vi "TP_Calculate.vi"(8 "error in (no error)":errorcluster, 10 "t":dbl=-1.0, 11 "TrapezoidalProfile in":refnum<class "TrapezoidalProfile.lvclass">) -> (0 "error out":errorcluster, 2 "Output":T1, 3 "TrapezoidalProfile out":refnum<class "TrapezoidalProfile.lvclass">)   [LabVIEW 2018, in "TrapezoidalProfile.lvclass"]
doc: "Calculate the correct position and velocity for the profile at a time <b>t</b> where the beginning of the profile was at time t = 0.\n<b>t</b> Time since the beginning of the profile."
uses:
  TrapezoidalProfile.lvclass
  State.ctl
  TrapezoidalProfile.lvclass/TrapezoidalProfile.ctl
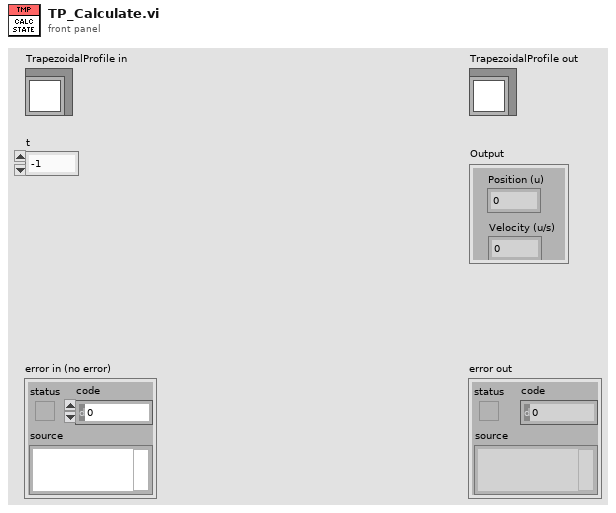
[diagram p1: front panel]
types:
  T1 = typedef "TrapezoidalProfile.lvclass/State.ctl" = cluster{"Position (u)":dbl, "Velocity (u/s)":dbl}
  T2 = typedef "TrapezoidalProfile.lvclass/Constraints.ctl" = cluster{"Max Velocity":dbl, "Max Accel":dbl}
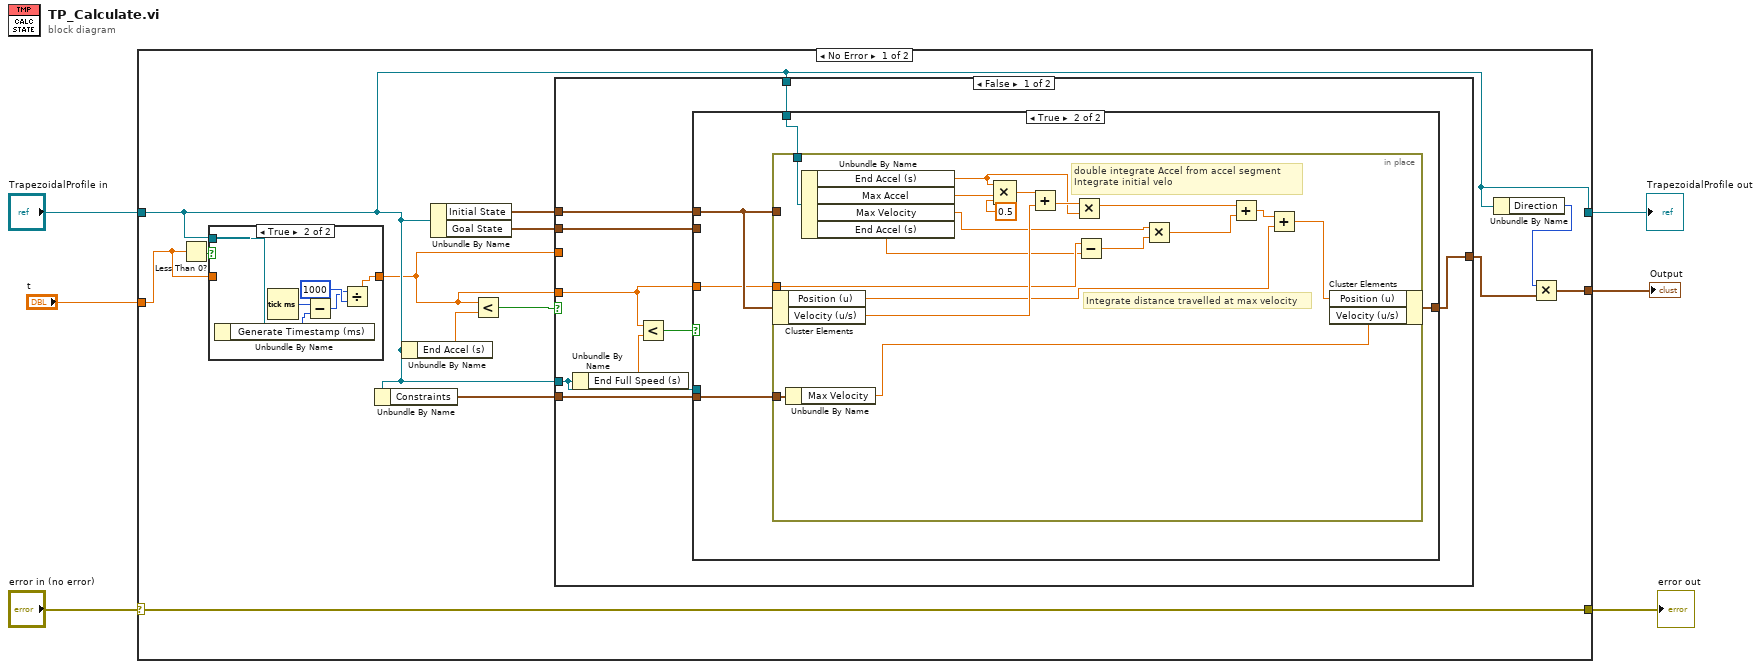
[diagram p0: block diagram]
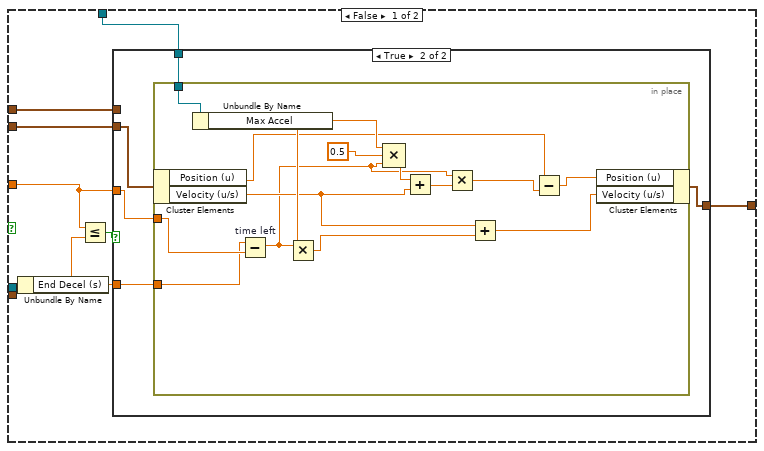
[diagram p3: hidden frame]
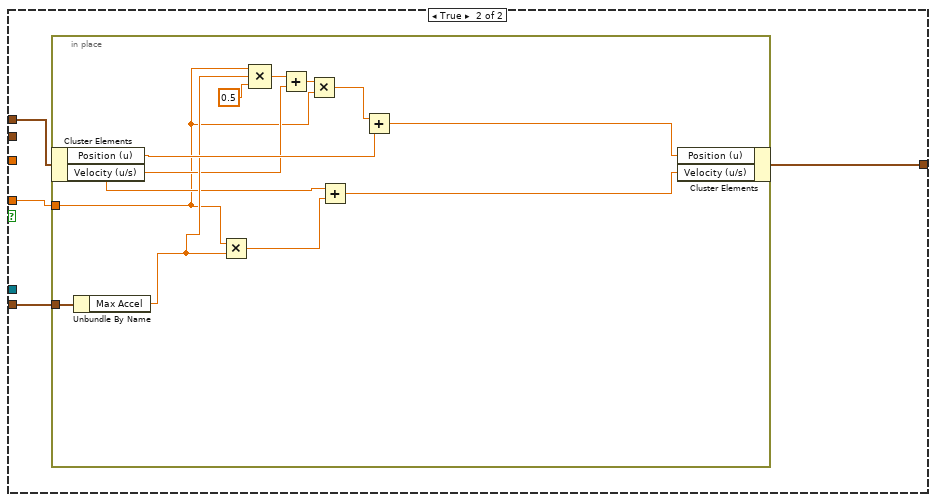
[diagram p5: hidden frame]
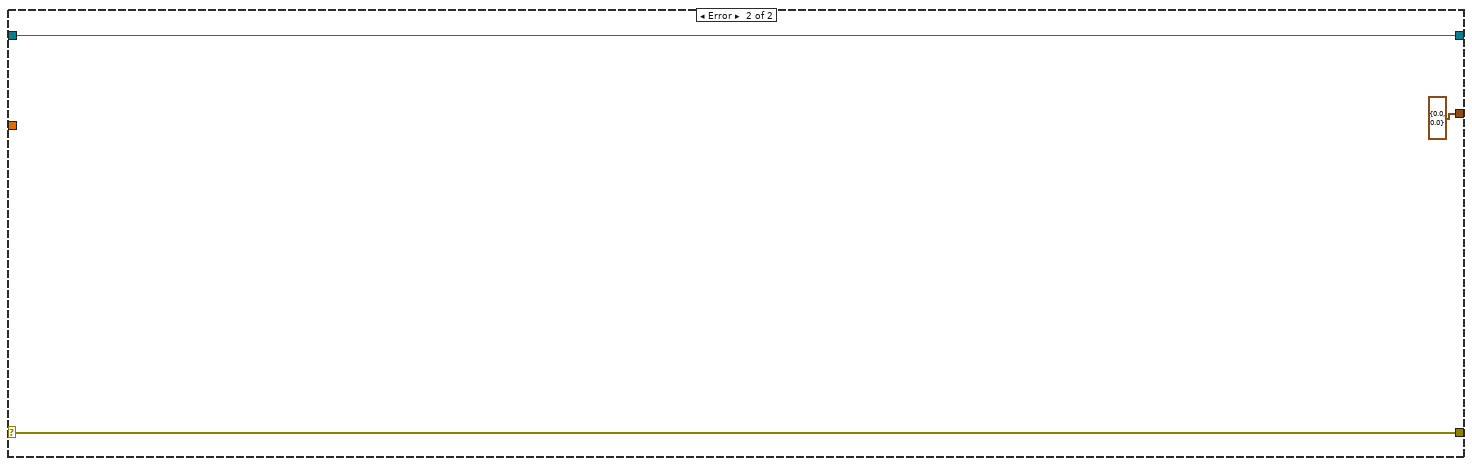
[diagram p6: hidden frame]
diagram:
  n1 = case shown="No Error" "error in (no error)" {
    selector: "error in (no error)" -> [w19 w105]
    tunnel: [w19 w105] -> w5
    tunnel: [w10 w104] -> w3
    tunnel: "TrapezoidalProfile in" -> [w10 w104]
    tunnel: "t" -> [w8 _]
    tunnel: [w11 T1 {"Position (u)"=0.0, "Velocity (u/s)"=0.0} ("Initial State")] -> w1
    frame No Error {
      n2 = Less Than 0?(x=w8) -> (x < 0?=w9:bool)
      n3 = case shown="True" w9 {
        tunnel: w10 -> [_ w26]
        tunnel: [w20 w23] -> w7
        tunnel: w8 -> [w20 _]
        frame False {
        }
        frame True {
          n4 = Unbundle By Name(w26) -> ("Generate Timestamp (ms)"=w24:u32)
          n5 = Tick Count (ms)() -> (millisecond timer value=w25:u32)
          n6 = Subtract(x=w25, y=w24) -> (x-y=w21:u32)
          n7 = Divide(x=w21, y=u32 1000 ("x")) -> (x/y=w23:dbl)
        }
      }
      n8 = Unbundle By Name(w10) -> ("Constraints"=w15:T2)
      n9 = Unbundle By Name(w10) -> ("End Accel (s)"=w18:dbl)
      n10 = Unbundle By Name(w10) -> ("Initial State"=w16:T1, "Goal State"=w14:T1)
      n11 = Less?(x=w7, y=w18) -> (x < y?=w17:bool)
      n12 = case shown="False" w17 {
        tunnel: w7 -> [_ _]
        tunnel: w16 -> [w33 w90]
        tunnel: w15 -> [w32 w89]
        tunnel: w7 -> [w31 w88]
        tunnel: [w28 w87] -> w12
        tunnel: w10 -> [w27 _]
        tunnel: w10 -> [w30 _]
        tunnel: w14 -> [w29 _]
        frame False {
          n13 = Unbundle By Name(w27) -> ("End Full Speed (s)"=w34:dbl)
          n14 = Less?(x=w31, y=w34) -> (x < y?=w35:bool)
          n15 = case shown="True" w35 {
            tunnel: w33 -> [w41 w67]
            tunnel: w32 -> [_ w68]
            tunnel: w31 -> [w37 w66]
            tunnel: w30 -> [w36 w65]
            tunnel: w29 -> [w43 _]
            tunnel: [w42 w64] -> w28
            tunnel: w27 -> [w39 _]
            frame False {
              n16 = Unbundle By Name(w39) -> ("End Decel (s)"=w38:dbl)
              n17 = Less Or Equal?(x=w37, y=w38) -> (x <= y?=w40:bool)
              n18 = case shown="True" w40 {
                tunnel: w43 -> [w44 w48]
                tunnel: [w44 w45] -> w42
                tunnel: w41 -> [_ _]
                tunnel: w38 -> [_ w49]
                tunnel: w37 -> [_ w47]
                tunnel: w36 -> [_ w46]
                frame False {
                }
                frame True {
                  n19 = in-place {
                    in-place-border: w49 -> [w62]
                    in-place-border: w47 -> [w63]
                    in-place-border: w46 -> [w61]
                    n20 = in-place-cluster #1(w48) -> ("Position (u)"=w50:dbl, "Velocity (u/s)"=w55:dbl)
                    n21 = Unbundle By Name(w61) -> ("Max Accel"=w58:dbl)
                    n22 = Subtract "time left"(x=w62, y=w63) -> (x-y=w53:dbl)
                    n23 = Multiply(x=w53, y=w58) -> (x*y=w60:dbl)
                    n24 = Compound Arithmetic op=MULTIPLY(w58, 0.5 ("value"), w53) -> (w56:dbl)
                    n25 = Add(x=w56, y=w55) -> (x+y=w54:dbl)
                    n26 = Multiply(x=w53, y=w54) -> (x*y=w51:dbl)
                    n27 = Add(x=w55, y=w60) -> (x+y=w59:dbl)
                    n28 = Subtract(x=w50, y=w51) -> (x-y=w52:dbl)
                    n29 = in-place-cluster #1("Position (u)"=w52, "Velocity (u/s)"=w59) -> (w45:T1)
                  }
                }
              }
            }
            frame True {
              n30 = in-place {
                in-place-border: w68 -> [w86]
                in-place-border: w67 -> [_]
                in-place-border: w66 -> [w77]
                in-place-border: w65 -> [w84]
                # "Integrate distance travelled at max velocity"
                # "double integrate Accel from accel segment\nIntegrate initial velo"
                n31 = in-place-cluster #2(w67) -> ("Position (u)"=w71:dbl, "Velocity (u/s)"=w81:dbl)
                n32 = Unbundle By Name(w86) -> ("Max Velocity"=w85:dbl)
                n33 = Unbundle By Name(w84) -> ("End Accel (s)"=w69:dbl, "Max Accel"=w79:dbl, "Max Velocity"=w78:dbl, "End Accel (s)"=w76:dbl)
                n34 = Compound Arithmetic op=MULTIPLY(w69, w79, 0.5 ("value")) -> (w82:dbl)
                n35 = Add(x=w82, y=w81) -> (x+y=w80:dbl)
                n36 = Multiply(x=w80, y=w69) -> (x*y=w74:dbl)
                n37 = Subtract(x=w77, y=w76) -> (x-y=w75:dbl)
                n38 = Multiply(x=w78, y=w75) -> (x*y=w73:dbl)
                n39 = Add(x=w74, y=w73) -> (x+y=w72:dbl)
                n40 = Add(x=w72, y=w71) -> (x+y=w70:dbl)
                n41 = in-place-cluster #2("Position (u)"=w70, "Velocity (u/s)"=w85) -> (w64:T1)
              }
            }
          }
        }
        frame True {
          n42 = in-place {
            in-place-border: w89 -> [w101]
            in-place-border: w88 -> [w92]
            n43 = in-place-cluster #3(w90) -> ("Position (u)"=w98:dbl, "Velocity (u/s)"=w94:dbl)
            n44 = Unbundle By Name(w101) -> ("Max Accel"=w97:dbl)
            n45 = Multiply(x=w92, y=w97) -> (x*y=w99:dbl)
            n46 = Compound Arithmetic op=MULTIPLY(w92, w97, 0.5 ("value")) -> (w95:dbl)
            n47 = Add(x=w95, y=w94) -> (x+y=w93:dbl)
            n48 = Multiply(x=w93, y=w92) -> (x*y=w91:dbl)
            n49 = Add(x=w94, y=w99) -> (x+y=w102:dbl)
            n50 = Add(x=w91, y=w98) -> (x+y=w100:dbl)
            n51 = in-place-cluster #3("Position (u)"=w100, "Velocity (u/s)"=w102) -> (w87:T1)
          }
        }
      }
      n52 = Unbundle By Name(w10) -> ("Direction"=w13:i32)
      n53 = Multiply(x=w13, y=w12) -> (x*y=w11:T1)
    }
    frame Error {
    }
  }
  "error out" <- w5
  "TrapezoidalProfile out" <- w3
  "Output" <- w1
